vi "SECoP_dataGetString.vi"(7 "Position":u32, 8 "error in (no error)":errorcluster, 10 "SECoP_dataPtr":T1 {"ptr64" format="%.0x"; "ptr32" format="%.0x"}, 11 "DLL path (in)":T2) -> (0 "error out":errorcluster, 2 "Value":string, 3 "DLL path (out)":T2)   [LabVIEW 2023, in "SECoP.lvlib"]
doc: "Call <b>\"SECoP_dataGetString.vi\"</b> to access the string value (SECoP_dataPtr).\n\n<b>DLL path</b> input and output of cluster from \"SECoP-Initialize.vi\"\n<b>SECoP_dataPtr</b> data to access\n<b>Position</b> points to a virtual flattened entry of the data type\n<b>Value</b> string value"
uses:
  SECoP.lvlib
  SECoP-libraries.ctl
  SECoP-data.ctl
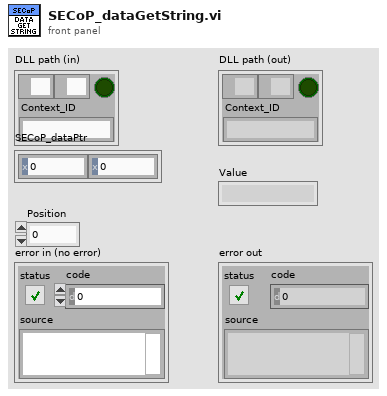
[diagram p1: front panel]
types:
  T1 = typedef "SECoP.lvlib/SECoP-data.ctl" = cluster{"ptr32":u32, "ptr64":u64}
  T2 = typedef "SECoP.lvlib/SECoP-libraries.ctl" = cluster{"serverDLL":path, "variantDLL":path, "cleanup_mode":bool, "Context_ID":string}
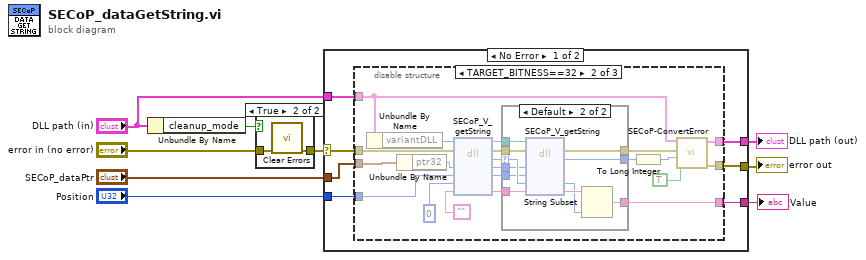
[diagram p0: block diagram]
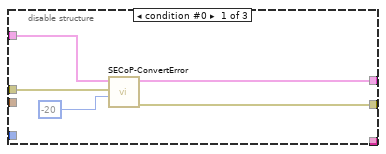
[diagram p3: hidden frame]
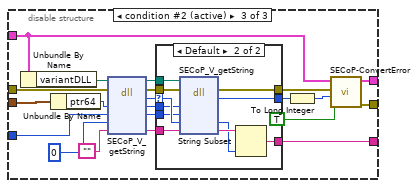
[diagram p5: hidden frame]
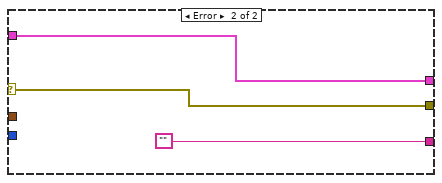
[diagram p7: hidden frame]
diagram:
  n1 = Unbundle By Name("DLL path (in)") -> ("cleanup_mode"=w7:bool)
  n2 = case shown="True" w7 {
    tunnel: "error in (no error)" -> [w10 w12]
    tunnel: [w10 w11] -> w5
    frame False {
    }
    frame True {
      n3 = call <vilib>:"Clear Errors.vi"("error in (no error)"=w12) -> ("error out"=w11:errorcluster)  [unwired: 5 in, 1 out]
    }
  }
  n4 = case shown="No Error" w5 {
    selector: w5 -> [w19 w96]
    tunnel: "DLL path (in)" -> [w13 w97]
    tunnel: [w15 w97] -> w9
    tunnel: [w16 w96] -> w8
    tunnel: "Position" -> [w18 _]
    tunnel: [w17 ""] -> w3
    tunnel: "SECoP_dataPtr" -> [w14 _]
    frame No Error {
      n5 = disable-structure shown="TARGET_BITNESS==32" {
        disable-tunnel: w19 -> [w21 w45 w80]
        disable-tunnel: w18 -> [_ w44 w79]
        disable-tunnel: [_ w35 w70] -> w17
        disable-tunnel: [w23 w29 w64] -> w16
        disable-tunnel: [w24 w30 w65] -> w15
        disable-tunnel: w14 -> [_ w42 w77]
        disable-tunnel: w13 -> [w22 w25 w60]
        frame condition #0 {
          n6 = call "SECoP-ConvertError.vi"("return code"=-20, "error in (no error)"=w21, "DLL path (in)"=w22) -> ("error out"=w23:errorcluster, "DLL path (out)"=w24:T2)  [unwired: 7 in]
        }
        frame condition #1 {
          n7 = Unbundle By Name(w25) -> ("variantDLL"=w26:path)
          n8 = Unbundle By Name(w42) -> ("ptr32"=w41:u32)
          n9 = dll-call lib="Z:/Praktische_Aufgaben/SECoP-LabVIEW2015/32bit/SECoP32.dll" fn="SECoP_V_getString"(path in=w26, error in=w45, "Data"=w41, "Position"=w44, "BufferSize"=u32 0, "Value"="") -> (path out=w38:path, error out=w37:errorcluster, "return type"=w39:u32, "Data"=w28:u32, "Position"=w27:u32, "Value"=w36:string)  [unwired: 2 in]
          n10 = case shown="Default" w39 {
            selector: w39 -> [w47 w56]
            tunnel: w38 -> [_ w59]
            tunnel: w37 -> [w48 w58]
            tunnel: [w48 w57] -> w31
            tunnel: [w47 w55] -> w32
            tunnel: w36 -> [w46 w54]
            tunnel: [w46 w51] -> w35
            tunnel: w28 -> [_ w50]
            tunnel: w27 -> [_ w49]
            frame 0 {
            }
            frame Default {
              n11 = dll-call lib="Z:/Praktische_Aufgaben/SECoP-LabVIEW2015/32bit/SECoP32.dll" fn="SECoP_V_getString"(path in=w59, error in=w58, "Data"=w50, "Position"=w49, "BufferSize"=w56, "Value"=w54) -> (error out=w57:errorcluster, "return type"=w55:u32, "BufferSize"=w52:u32, "Value"=w53:string)  [unwired: 3 in, 1 out]
              n12 = String Subset(string=w53, length (rest)=w52) -> (substring=w51:string)  [unwired: 1 in]
            }
          }
          n13 = To Long Integer(number=w32) -> (32bit integer=w33:i32)
          n14 = call "SECoP-ConvertError.vi"("return is boolean"=TRUE, "return code"=w33, "error in (no error)"=w31, "DLL path (in)"=w25) -> ("error out"=w29:errorcluster, "DLL path (out)"=w30:T2)  [unwired: 6 in]
        }
        frame condition #2 (active) {
          n15 = Unbundle By Name(w60) -> ("variantDLL"=w61:path)
          n16 = Unbundle By Name(w77) -> ("ptr64"=w76:u64)
          n17 = dll-call lib="Z:/Praktische_Aufgaben/SECoP-LabVIEW2015/32bit/SECoP32.dll" fn="SECoP_V_getString"(path in=w61, error in=w80, "Data"=w76, "Position"=w79, "BufferSize"=u32 0, "Value"="") -> (path out=w73:path, error out=w72:errorcluster, "return type"=w74:u32, "Data"=w63:u64, "Position"=w62:u32, "Value"=w71:string)  [unwired: 2 in]
          n18 = case shown="Default" w74 {
            selector: w74 -> [w82 w91]
            tunnel: w73 -> [_ w94]
            tunnel: w72 -> [w83 w93]
            tunnel: [w83 w92] -> w66
            tunnel: [w82 w90] -> w67
            tunnel: w71 -> [w81 w89]
            tunnel: [w81 w86] -> w70
            tunnel: w63 -> [_ w85]
            tunnel: w62 -> [_ w84]
            frame 0 {
            }
            frame Default {
              n19 = dll-call lib="Z:/Praktische_Aufgaben/SECoP-LabVIEW2015/32bit/SECoP32.dll" fn="SECoP_V_getString"(path in=w94, error in=w93, "Data"=w85, "Position"=w84, "BufferSize"=w91, "Value"=w89) -> (error out=w92:errorcluster, "return type"=w90:u32, "BufferSize"=w87:u32, "Value"=w88:string)  [unwired: 3 in, 1 out]
              n20 = String Subset(string=w88, length (rest)=w87) -> (substring=w86:string)  [unwired: 1 in]
            }
          }
          n21 = To Long Integer(number=w67) -> (32bit integer=w68:i32)
          n22 = call "SECoP-ConvertError.vi"("return is boolean"=TRUE, "return code"=w68, "error in (no error)"=w66, "DLL path (in)"=w60) -> ("error out"=w64:errorcluster, "DLL path (out)"=w65:T2)  [unwired: 6 in]
        }
      }
    }
    frame Error {
    }
  }
  "DLL path (out)" <- w9
  "error out" <- w8
  "Value" <- w3
